vi "VCS Set Position Profile.vi"(8 "error in (no error)":errorcluster, 10 "position profile":T1, 11 "axis in":cluster{"keyHandle":u32, "nodeId":u16}={"keyHandle"=0, "nodeId"=1}) -> (0 "error out":errorcluster, 3 "axis out":cluster{"keyHandle":u32, "nodeId":u16}={"keyHandle"=0, "nodeId"=1})   [LabVIEW 2018]
doc: "<B>VCS Set Position Profile</B> writes the position profile parameters."
uses:
  Resources/EposCmd.dll
  Resources/EposCmd64.dll
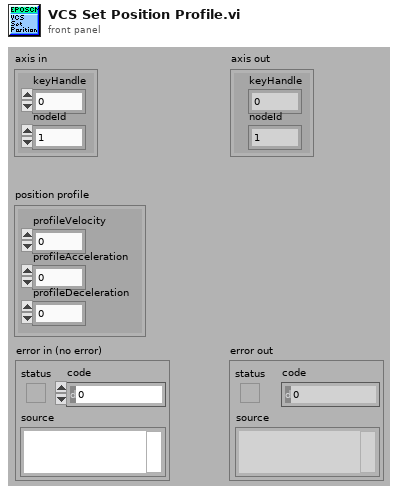
[diagram p1: front panel]
types:
  T1 = cluster{"profileVelocity":u32, "profileAcceleration":u32, "profileDeceleration":u32}
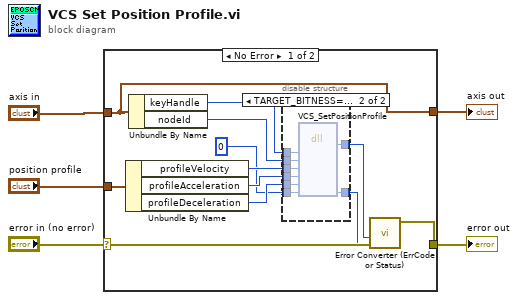
[diagram p0: block diagram]
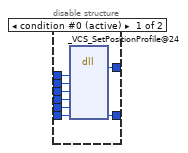
[diagram p2: hidden frame]
diagram:
  n1 = case shown="No Error" "error in (no error)" {
    selector: "error in (no error)" -> [w17 w35]
    tunnel: [w16 w35] -> w4
    tunnel: "axis in" -> [w7 w34]
    tunnel: "position profile" -> [w12 _]
    tunnel: [w7 w34] -> w1
    frame No Error {
      n2 = Unbundle By Name(w12) -> ("profileVelocity"=w11:u32, "profileAcceleration"=w10:u32, "profileDeceleration"=w9:u32)
      n3 = Unbundle By Name(w7) -> ("keyHandle"=w14:u32, "nodeId"=w13:u16)
      n4 = disable-structure shown="TARGET_BITNESS==64" {
        disable-tunnel: [w25 w33] -> w15
        disable-tunnel: w14 -> [w24 w32]
        disable-tunnel: w13 -> [w23 w31]
        disable-tunnel: w11 -> [w22 w30]
        disable-tunnel: w10 -> [w21 w29]
        disable-tunnel: w9 -> [w20 w28]
        disable-tunnel: u32 0 ("pErrorCode") -> [w19 w27]
        disable-tunnel: [w18 w26] -> w6
        frame condition #0 (active) {
          n5 = dll-call lib="C:/Projeto em LabVIEW/EPOS-LabVIEW-Instrument-Driver-En/LabVIEW/maxon EPOS/Resources/EposCmd.*" fn="_VCS_SetPositionProfile@24"("KeyHandle"=w24, "NodeId"=w23, "ProfileVelocity"=w22, "ProfileAcceleration"=w21, "ProfileDeceleration"=w20, "pErrorCode"=w19) -> (w18:i32, "pErrorCode"=w25:u32)  [unwired: 8 in, 2 out]
        }
        frame condition #1 {
          n6 = dll-call lib="C:/setup/Resources/EposCmd64.*" fn="VCS_SetPositionProfile" ("EposCmd.dll:_VCS_SetPositionProfile@24")("KeyHandle"=w32, "NodeId"=w31, "ProfileVelocity"=w30, "ProfileAcceleration"=w29, "ProfileDeceleration"=w28, "pErrorCode"=w27) -> ("Rückgabetyp"=w26:i32, "pErrorCode"=w33:u32)  [unwired: 8 in, 2 out]
        }
      }
      n7 = call "Error Converter (ErrCode or Status).vi"("error code"=w15, "return type"=w6, "error in (no error)"=w17) -> ("error out"=w16:errorcluster)  [unwired: 7 in]
    }
    frame Error {
    }
  }
  "error out" <- w4
  "axis out" <- w1
